vi "Clear (No Check).vi"(8 "error in (no error)":errorcluster, 9 "offset (0)":u64 format="%d bytes", 10 "size":u64 format="%d bytes", 11 "Pointer in":refnum<class "Pointer.lvclass">) -> (0 "error out":errorcluster, 3 "Pointer out":refnum<class "Pointer.lvclass">)   [LabVIEW 2027, in "Memory Manager.lvlib" / "Pointer.lvclass"]
doc: "Sets the subset of bytes specified by <b>offset</b> and <b>length</b> within the provided <b>pointer</b> to zero.\n\n<b>Note:</b> This VI is <b>unsafe</b>, meaning it does not performs null pointer and bounds checks to prevent invaid memory access. Invalid arguments provided to this method can crash or corrupt LabVIEW memory."
uses:
  Pointer.lvclass
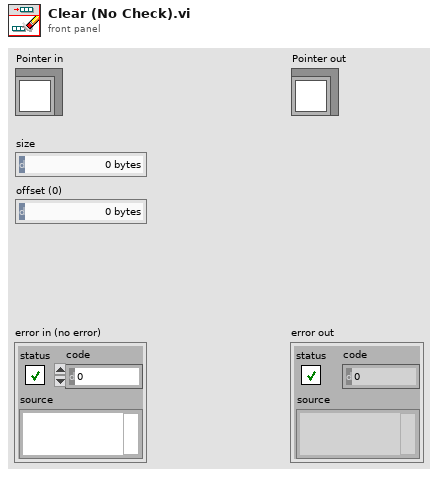
[diagram p1: front panel]
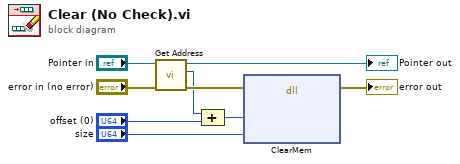
[diagram p0: block diagram]
diagram:
  n1 = call "Get Address.vi"("Pointer in"="Pointer in") -> ("address"=w5:u64, "Pointer out"=→"Pointer out":refnum<class "Pointer.lvclass">)  [unwired: 9 in]
  n2 = Compound Arithmetic op=ADD(w5, "offset (0)") -> (w4:u64)
  n3 = dll-call lib="LabVIEW" fn="ClearMem"(error in="error in (no error)", "pointer"=w4, "size"="size") -> (error out=→"error out":errorcluster)  [unwired: 5 in, 1 out]
